vi "SMBUS Process Call.vi"(4 "WithPEC":u8, 5 "pReadData":u16[](array[numeric])=array[4097 elements], 6 "WriteData":u16, 7 "CommandCode":u8, 9 "SlaveAddr":i16, 10 "IICIndex":i32, 11 "DevHandle":i32) -> (2 "function return":i32, 3 "pReadData out":u16[](array[numeric]))   [LabVIEW 2010, in "usb2iic.lvlib"]
doc: "int WINAPI SMBUS_ProcessCall(int DevHandle,int IICIndex,short SlaveAddr,unsigned char CommandCode, unsigned short WriteData, unsigned short *pReadData,unsigned char WithPEC);"
uses:
  usb2iic.lvlib
  USB2XXX.dll
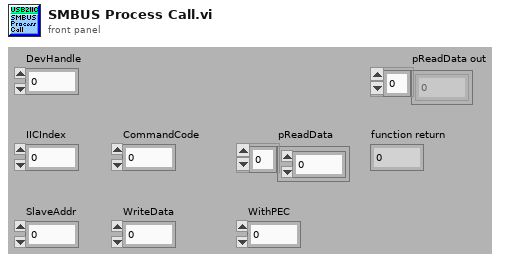
[diagram p1: front panel]
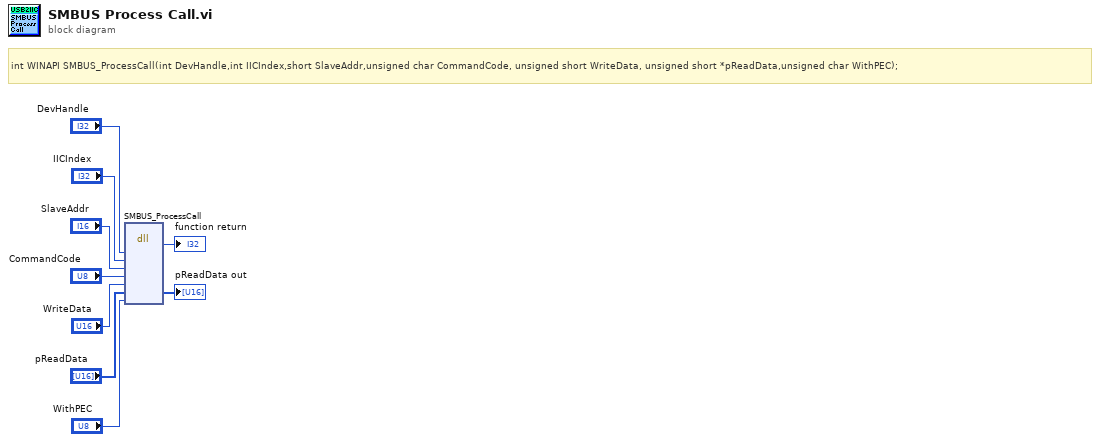
[diagram p0: block diagram]
diagram:
  # "int WINAPI SMBUS_ProcessCall(int DevHandle,int IICIndex,short SlaveAddr,unsigned char CommandCode, unsigned short WriteData, unsigned short *pReadData,unsigned char WithPEC);"
  n1 = dll-call lib="G:/OtherWork/USB2XXX_Example/trunk/Labview/PublicFiles/USB2XXX.*" fn="SMBUS_ProcessCall"("DevHandle"="DevHandle", "IICIndex"="IICIndex", "SlaveAddr"="SlaveAddr", "CommandCode"="CommandCode", "WriteData"="WriteData", "pReadData"="pReadData", "WithPEC"="WithPEC") -> (→"function return":i32, "pReadData"=→"pReadData out":u16[])  [unwired: 9 in, 2 out]
